vi "pH电极校准.vi"() -> ()   [LabVIEW 2016, in "斯坦道多参数.lvlib"]
uses:
  <vilib>/Utility/miscctls.llb/LVPointTypeDef.ctl
  <vilib>/Analysis/NI_AALBase.lvlib
panel:
  in  "刷新按钮":bool
  out "第三点信号值":dbl
  out "第二点信号值":dbl
  out "第一点信号值":dbl
  out "温度":dbl format="%#.2f"
  out "通讯状态":string
  out "电极状态标志":u16(ring) items=["OK", "第一点校正通过", "第二点校正通过", "校正失败,电极零点超出范围", "校正失败,电极斜率超出范围", "第三点校正通过"]
  in  "三点标液3":u16(ring)=6 caption="标液3" items=["TECH4.00", "TECH7.00", "TECH10.00", "NIST1.68", "NIST4.01", "NIST6.86", "NIST9.18", "NIST12.68"]
  in  "三点标液2":u16(ring)=5 caption="标液2" items=["TECH4.00", "TECH7.00", "TECH10.00", "NIST1.68", "NIST4.01", "NIST6.86", "NIST9.18", "NIST12.68"]
  in  "三点标液1":u16(ring)=4 caption="标液1" items=["TECH4.00", "TECH7.00", "TECH10.00", "NIST1.68", "NIST4.01", "NIST6.86", "NIST9.18", "NIST12.68"]
  out "第三点校准值":dbl
  in  "校准停止":bool
  in  "校准启动":bool
  out "第二点校准值":dbl
  out "第一点校准值":dbl
  out "提示":string
  in  "校准模式":u16(ring) items=["两点校准", "单点校准", "三点校准"]
  out "最小值":sgl format="%#.2f"
  out "最大值":sgl format="%#.2f"
  out "变异系数":dbl format="%#.6f"
  out "standard deviation":dbl caption="标准差" format="%#.2f"
  out "mean":dbl caption="均值" format="%#.2f"
  out "波形图表":dbl(graph) caption="历史曲线"
  out "当前检测值":dbl caption="测量值" format="%#.2f"
  out "标液2":dbl
  out "标液1":dbl
  out "当前信号值":dbl caption="信号值" format="%#.2f"
  out "偏移值补偿":dbl caption="pH偏移修正值" format="%#.2f"
  out "电极斜率":dbl format="%#.6f"
  out "电极零点":dbl format="%#.6f"
  # "酸碱度电极设定"
  # "℃"
  # "mV"
  # "mV"
  # "%"
  # "请选择校准模式:"
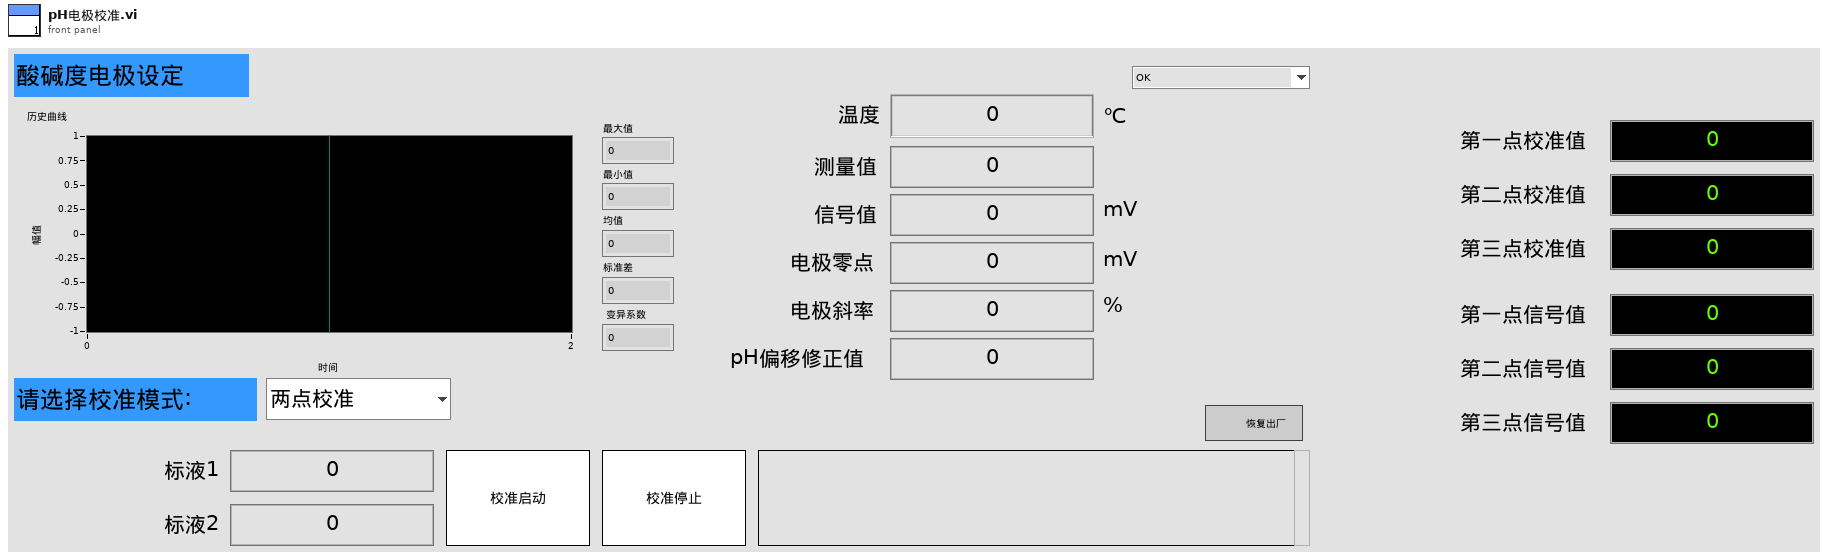
[diagram p1: front panel]
types:
  T1 = typedef "LVPointTypeDef.ctl" = cluster{"Horizontal":i16, "Vertical":i16}
  T2 = cluster{"电极状态标志":u16, "电极型号标志":u16, "酸碱度测量值":sgl, "温度测量值":sgl, "酸碱度信号值":sgl, "温度信号值":sgl, "酸碱度偏移修正值":sgl, "温度偏移修正值":sgl, "手动温度补偿值":sgl, "酸碱度电极零点":sgl, "酸碱度电极斜率":sgl, "第1点标准值记录":sgl, "第1点信号值记录":sgl, "第1点温度值记录":sgl, "第2点标准值记录":sgl, "第2点信号值记录":sgl, "第2点温度值记录":sgl, "命令滤波设定":u16, "温度模式":enum16{"ATC", "MTC"}, "生产批次":u16, "电极序号":u16, "串口地址":u16, "串口波特率":enum16{"9600", "19200", "115200"}, "串口校验位":enum16{"NONE", "ODD", "EVEN"}, "串口停止位":enum16{"1bit", "2bit"}, "第一点标准值":sgl, "第二点标准值":sgl}
  T3 = enum8{"Enabled", "Disabled", "Disabled and Grayed Out"}
  T4 = cluster{"ph":bool, "DO":bool, "Cond":bool, "Turb":bool, "叶绿素a":bool, "藻密度":bool, "ORP":bool}
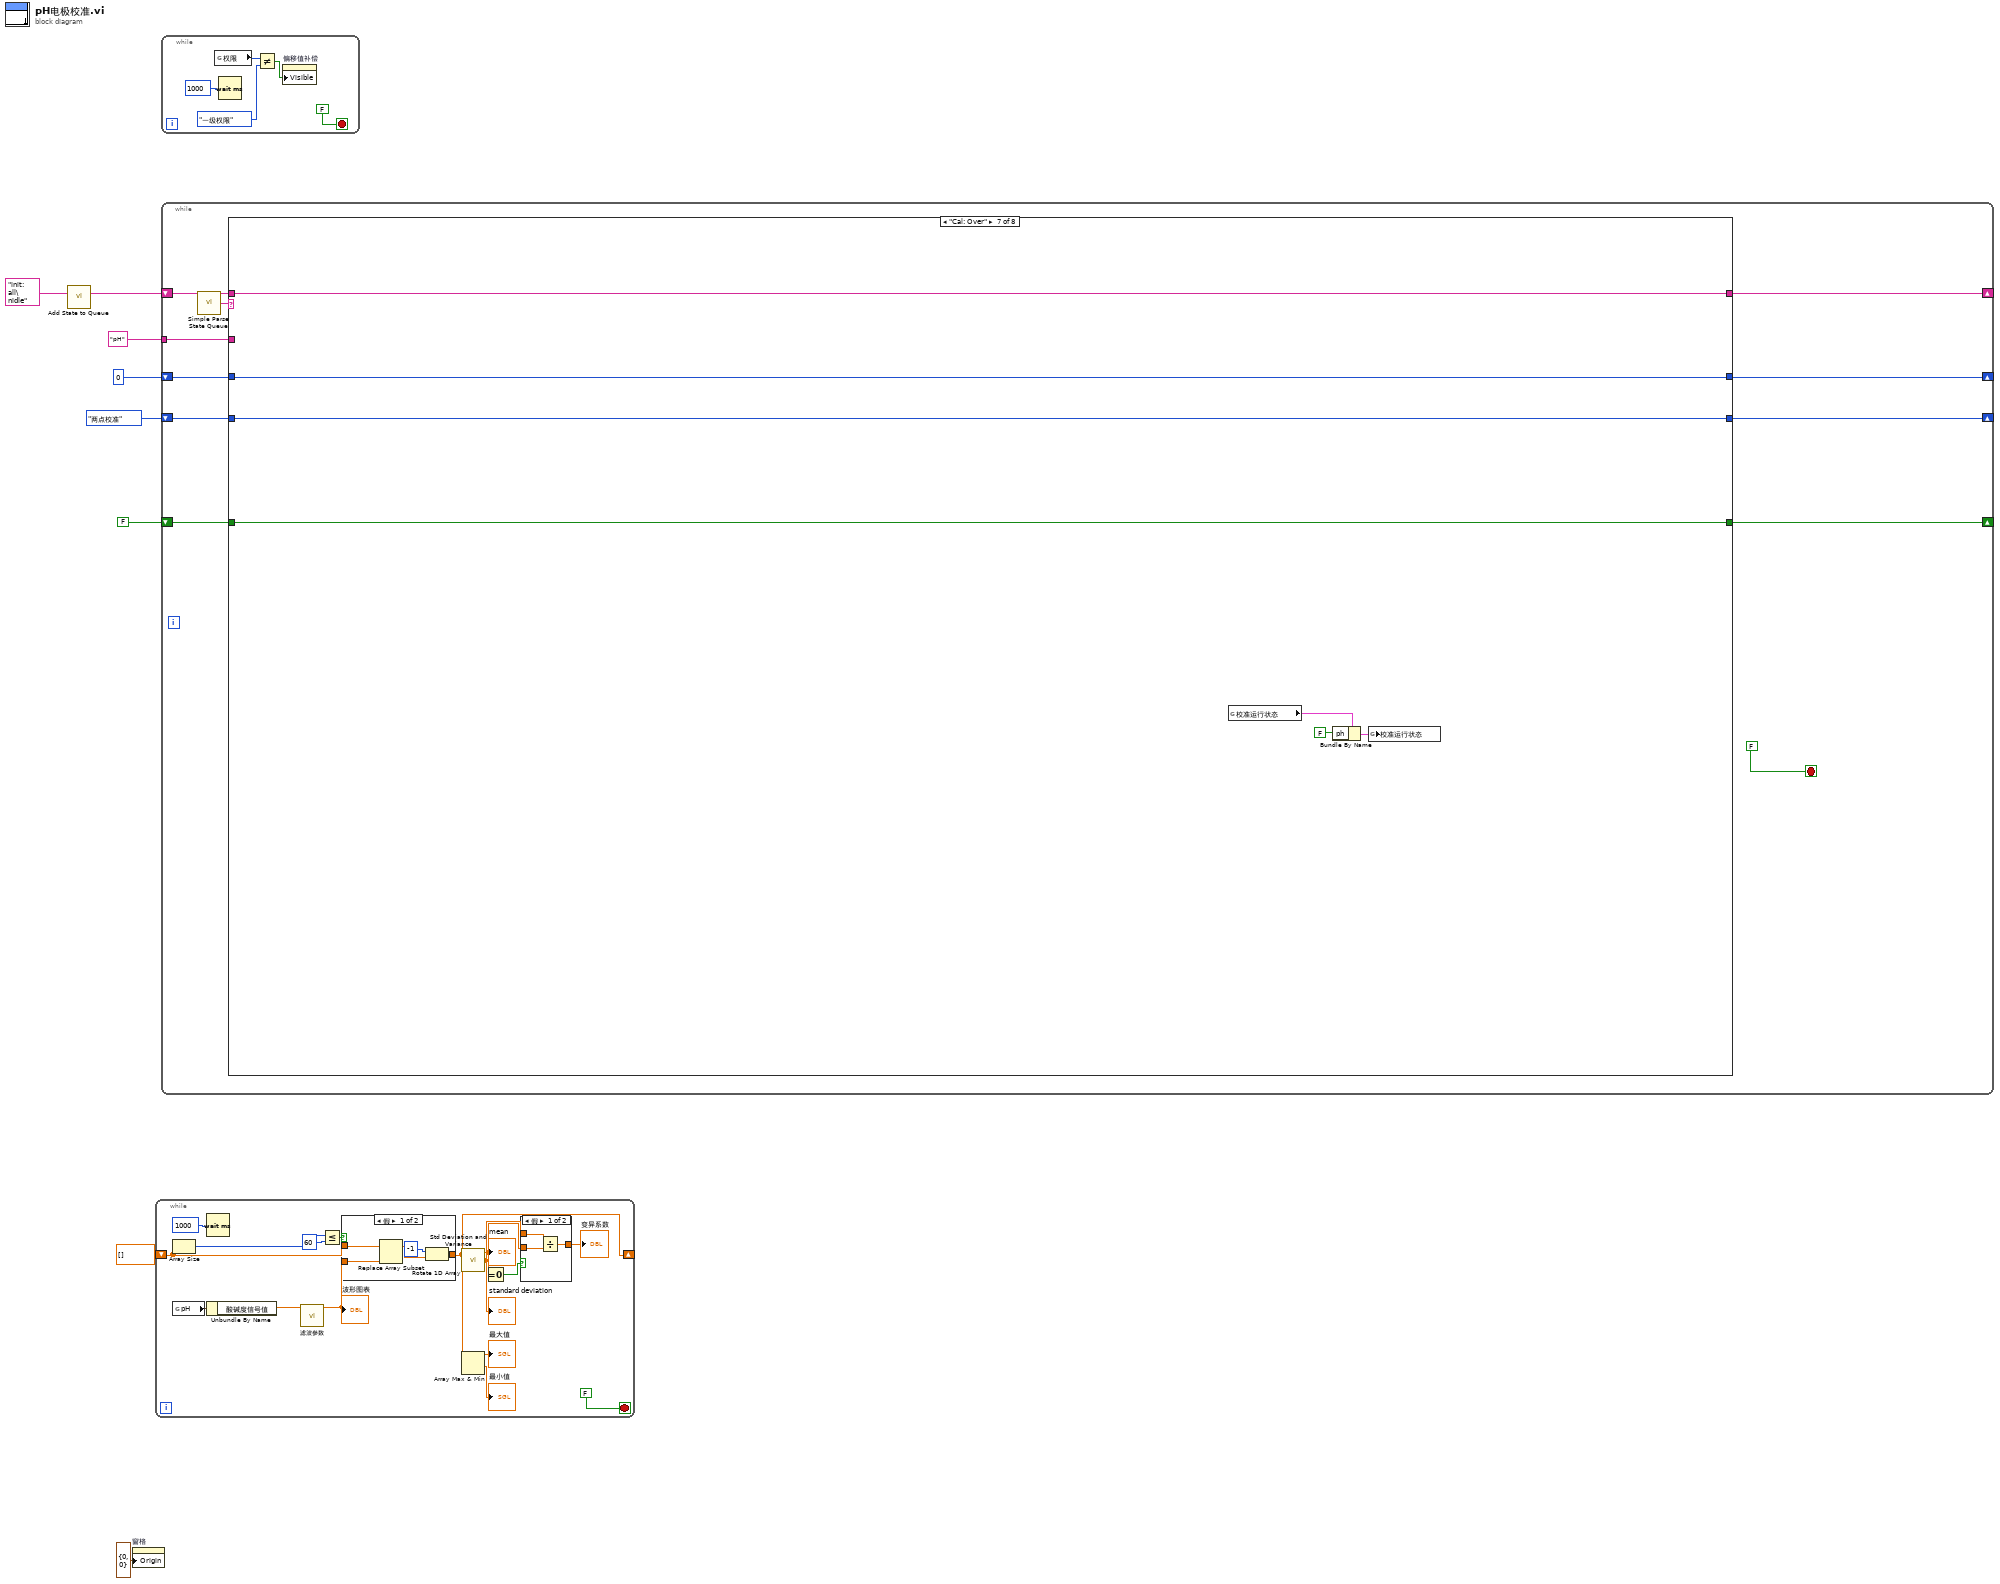
[diagram p0: block diagram]
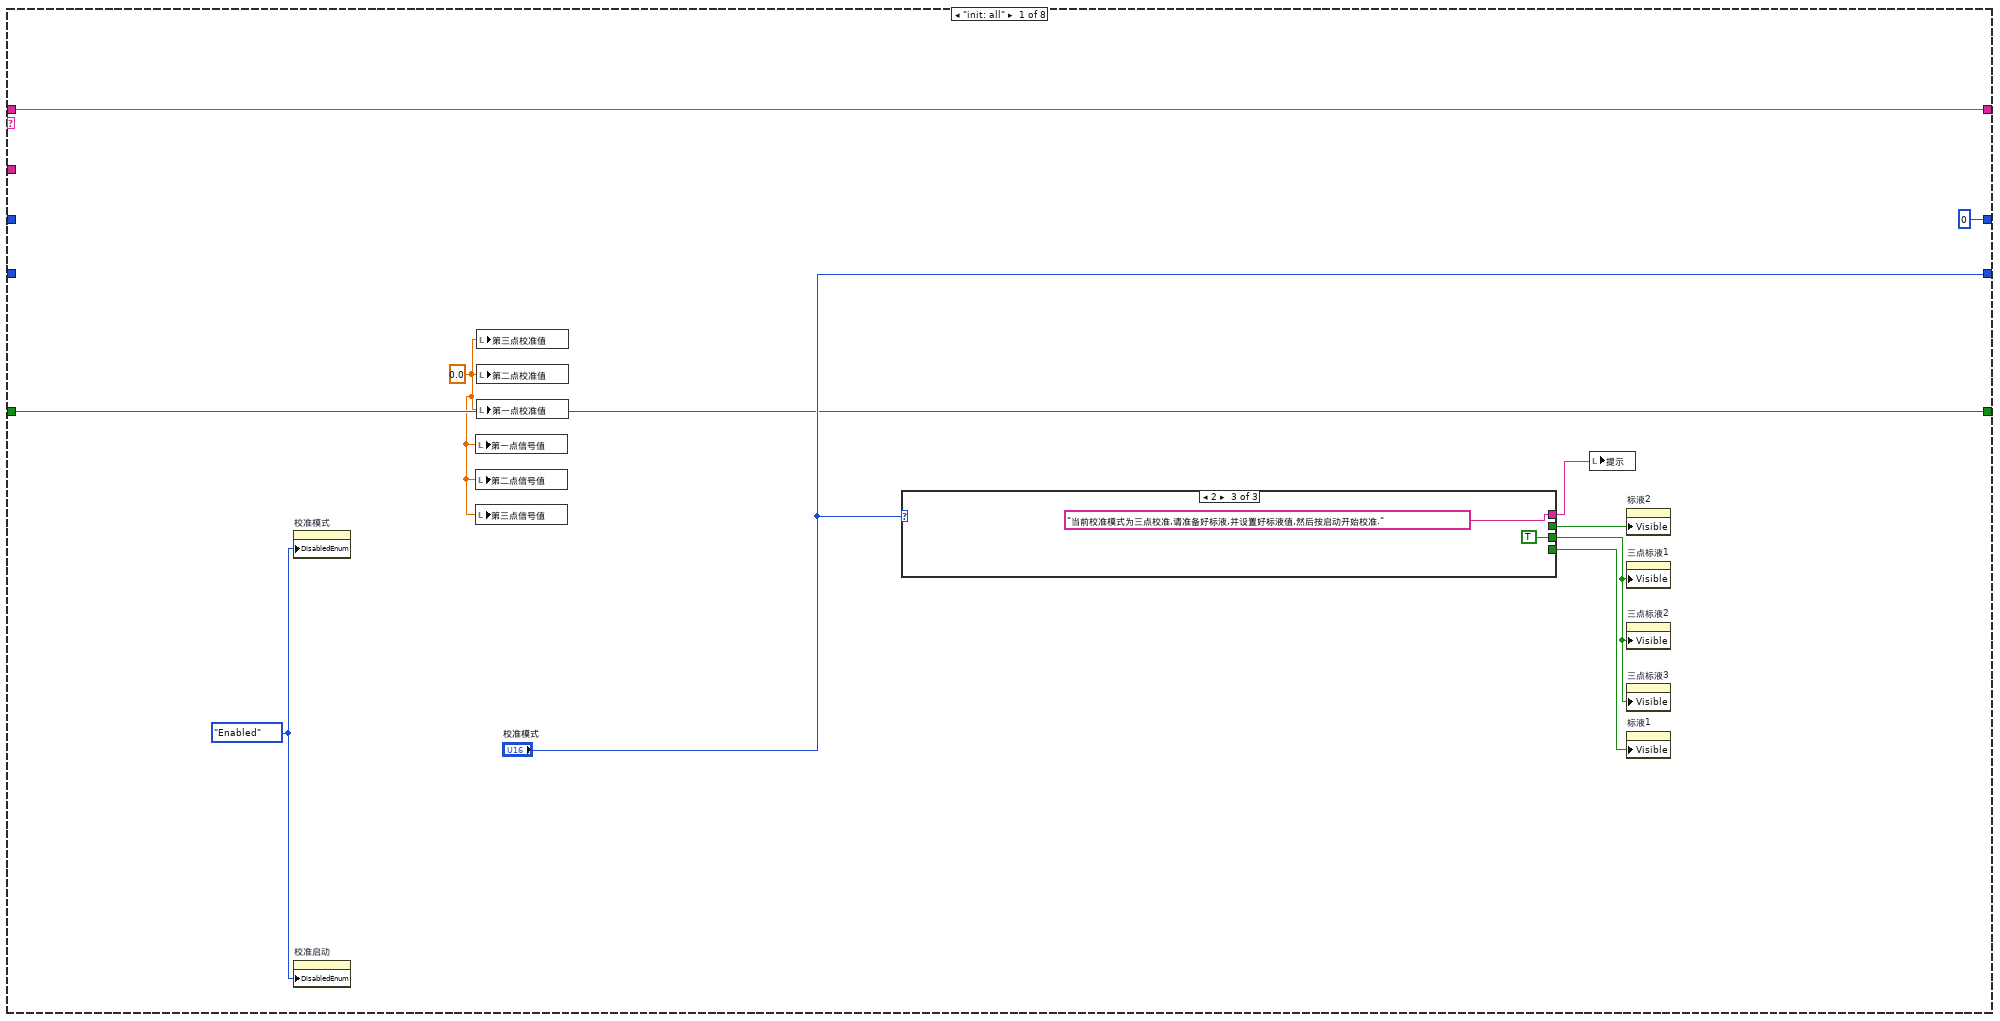
[diagram p2: hidden frame]
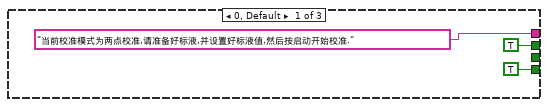
[diagram p3: hidden frame]
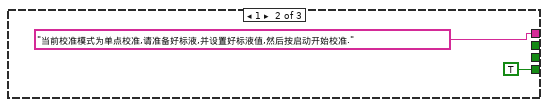
[diagram p4: hidden frame]
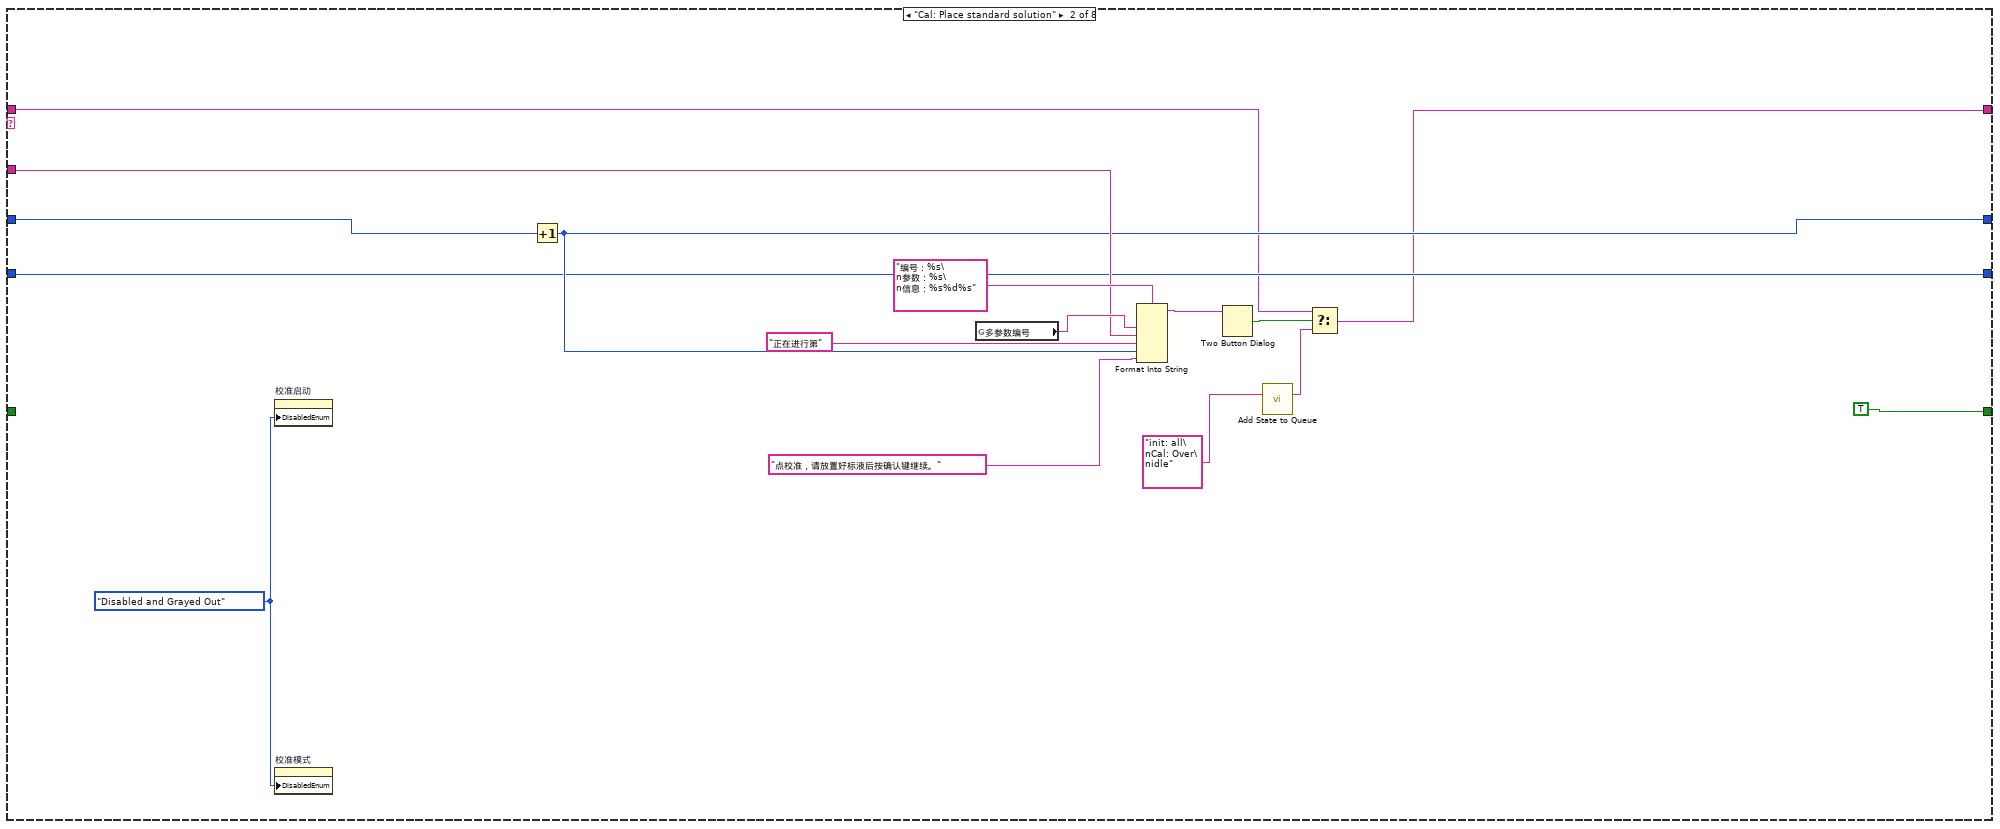
[diagram p5: hidden frame]
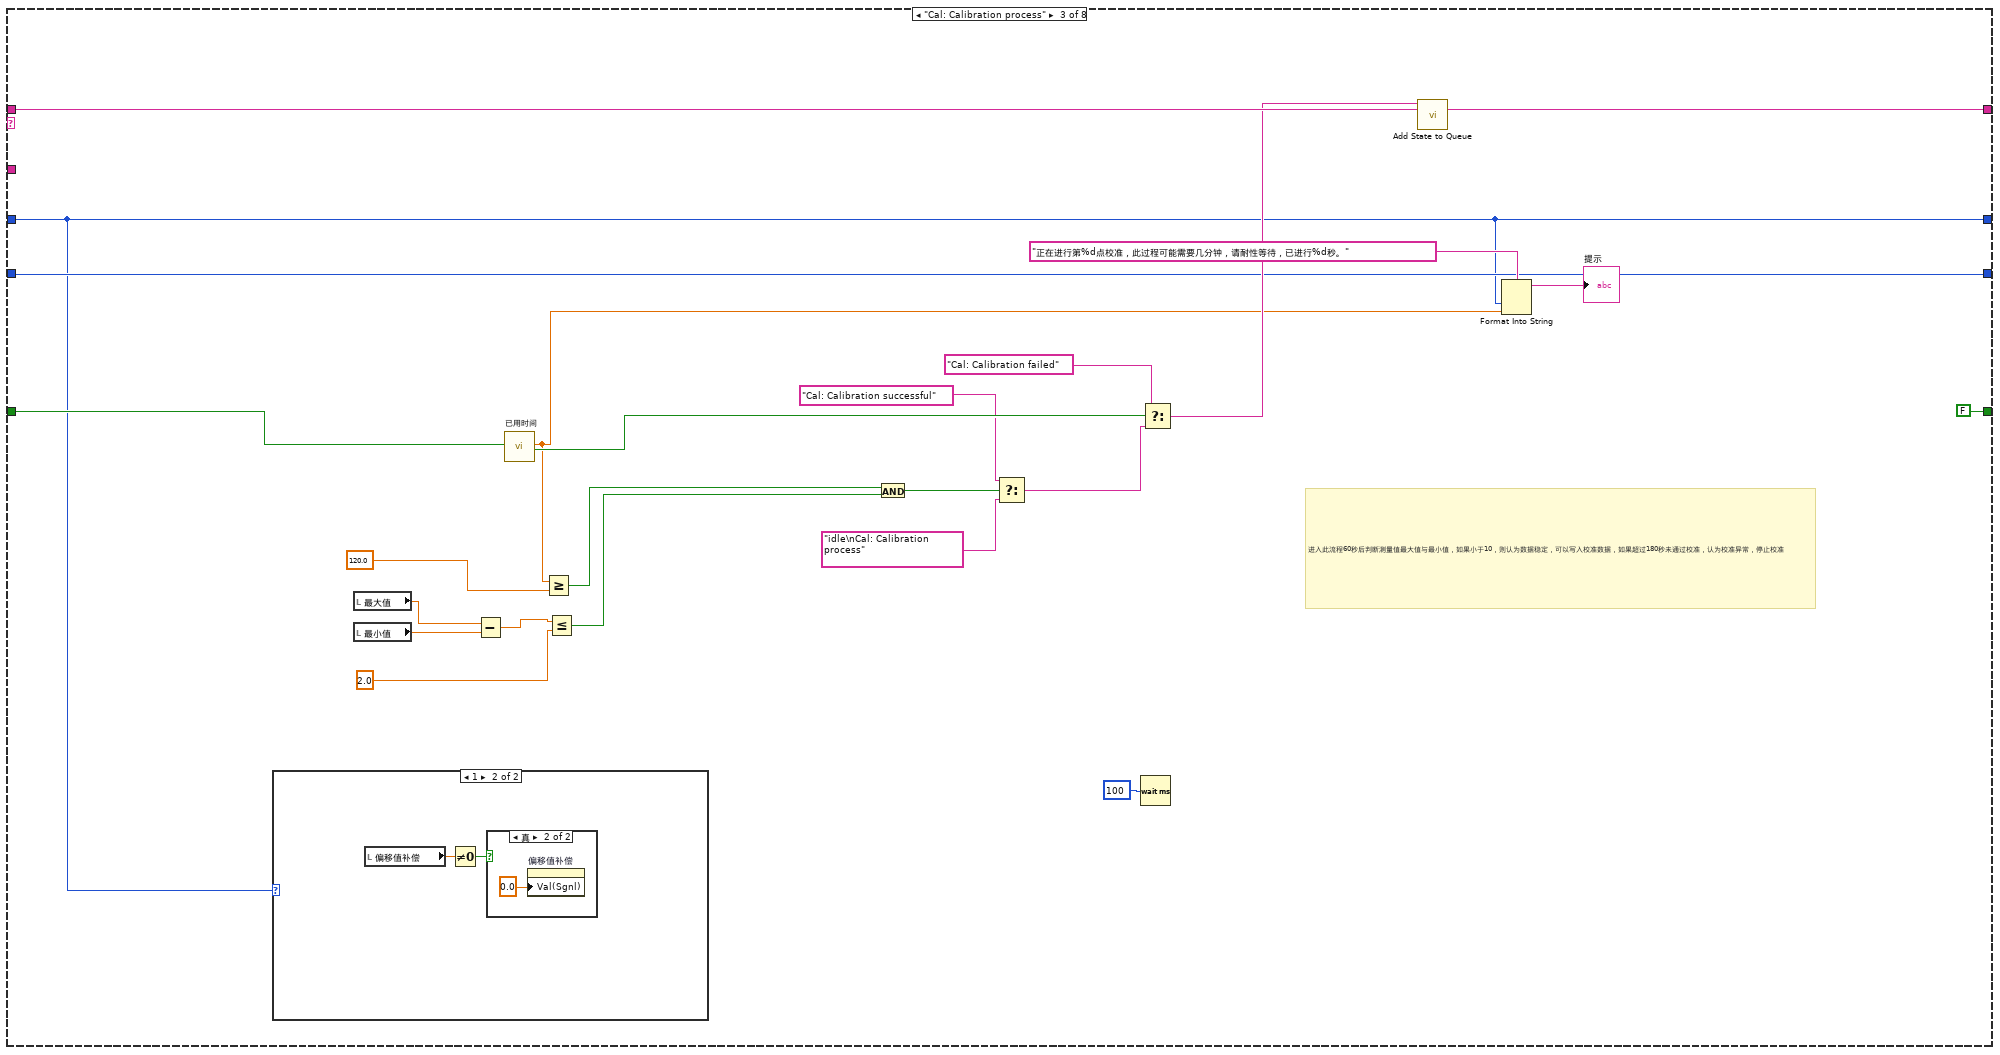
[diagram p6: hidden frame]
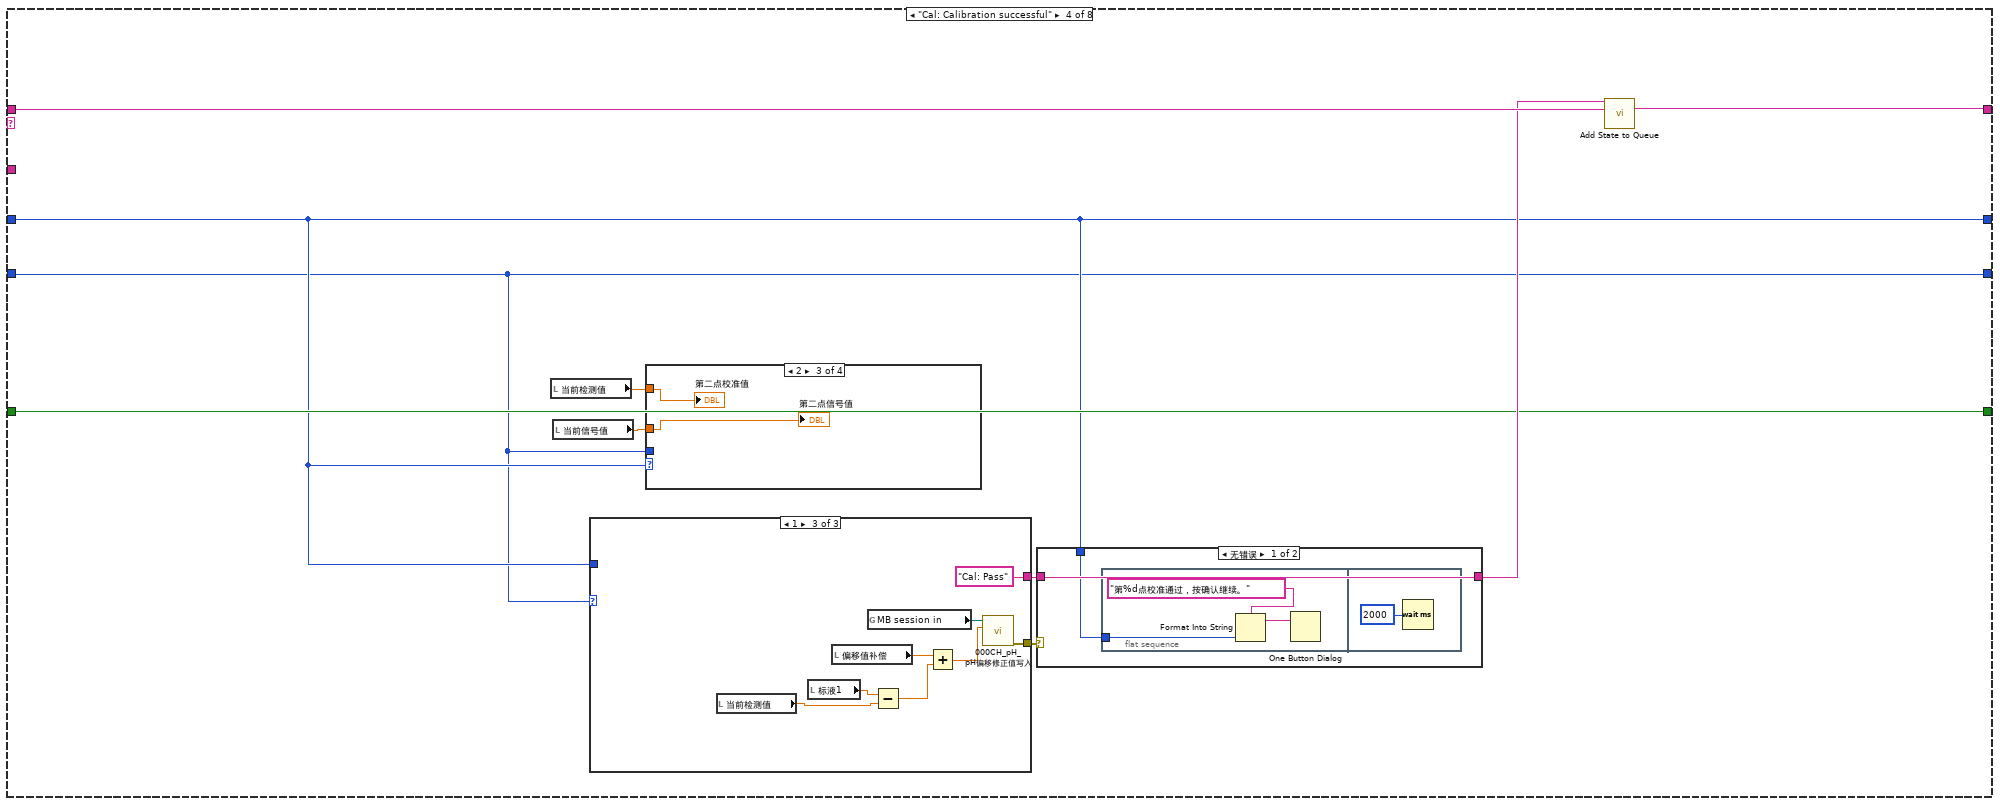
[diagram p9: hidden frame]
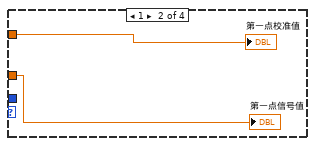
[diagram p11: hidden frame]
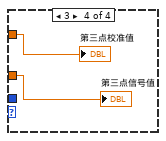
[diagram p12: hidden frame]
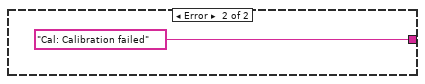
[diagram p13: hidden frame]
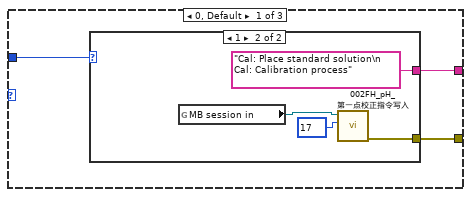
[diagram p14: hidden frame]
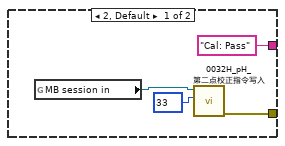
[diagram p15: hidden frame]
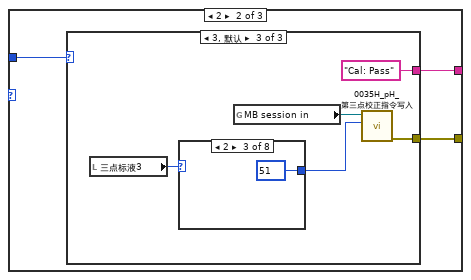
[diagram p16: hidden frame]
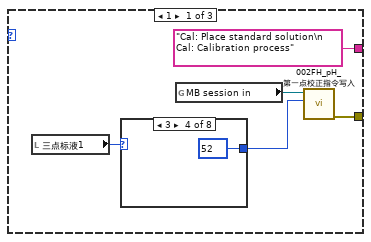
[diagram p17: hidden frame]
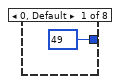
[diagram p18: hidden frame]
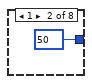
[diagram p19: hidden frame]
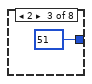
[diagram p20: hidden frame]
diagram:
  n1 = call "Add State to Queue.vi"("State(s) In (\"\")"="init: all\nidle" ("State(s) In (\"\")")) -> ("States Out"=w5:string)  [unwired: 14 in]
  n2 = property on="窗格" class="Pane"("Origin"=T1 {"Horizontal"=0, "Vertical"=0} ("原点")) -> ()  [unwired: 2 in, 2 out]
  n3 = while {
    shift-right: [w16] -> _
    shift-left: sgl[] [] -> [w20]
    stop <- FALSE stop-if-true
    n4 = Array Size(array=w20) -> (size(s)=w22:i32)
    n5 = global read "国弘过程全局变量.vi" "pH"() -> (w17:T2)
    n6 = Wait (ms)(milliseconds to wait=u32 1000 ("等待时间（毫秒）")) -> ()  [unwired: 1 out]
    n7 = Unbundle By Name(w17) -> ("酸碱度信号值"=w10:sgl)
    n8 = call "滤波参数.vi"("x"=w10) -> ("mode"=w9:dbl)  [unwired: 10 in]
    "波形图表" <- w9
    n9 = Less Or Equal?(x=w22, y=60) -> (x <= y?=w21:bool)
    n10 = case shown="假" w21 {
      tunnel: w20 -> [w32 w35]
      tunnel: w9 -> [w30 w34]
      tunnel: [w28 w33] -> w16
      frame False {
        n11 = Replace Array Subset(array=w32, new element=w30) -> (w31:sgl[])  [unwired: 1 in]
        n12 = Rotate 1D Array(1:w31, 2:-1 ("n")) -> (0:w28:sgl[])
      }
      frame True {
        n13 = Insert Into Array(array=w35, new element=w34) -> (w33:sgl[])  [unwired: 1 in]
      }
    }
    n14 = call <vilib>:"Std Deviation and Variance.vi"("X"=w16) -> ("mean"=w12:dbl, "standard deviation"=w11:dbl)  [unwired: 1 in, 1 out]
    "mean" <- w12
    "standard deviation" <- w11
    n15 = Array Max & Min(array=w16) -> (max value=→"最大值":sgl, min value=→"最小值":sgl)  [unwired: 2 out]
    n16 = Equal To 0?(x=w12) -> (x = 0?=w19:bool)
    n17 = case shown="假" w19 {
      tunnel: w11 -> [w27 _]
      tunnel: [w26 _] -> w13
      tunnel: w12 -> [w25 _]
      frame False {
        n18 = Divide(x=w27, y=w25) -> (x/y=w26:dbl)
      }
      frame True {
      }
    }
    "变异系数" <- w13
  }
  n19 = while {
    shift-right: [w43] -> _
    shift-left: w5 -> [w47]
    shift-right: [w40] -> _
    shift-left: 0 -> [w42]
    tunnel: "pH" ("State(s) In (\"\")") -> [w41]
    shift-right: [w38] -> _
    shift-left: enum16{"两点校准", "单点校准", "三点校准"}."两点校准" ("校准模式") -> [w39]
    shift-right: [w36] -> _
    shift-left: FALSE -> [w37]
    stop <- FALSE stop-if-true
    n20 = call "Simple Parse State Queue.vi"("State Queue"=w47) -> ("Remain States"=w44:string, "Next State"=w45:string)  [unwired: 13 in]
    n21 = case shown="\"Cal: Over\"" w45 {
      tunnel: w44 -> [w57 w67 w99 w115 _ _ w260 w270]
      tunnel: [w57 w66 w98 w114 w199 w206 w260 w269] -> w43
      tunnel: w42 -> [_ w76 w82 w109 w202 w215 w259 w267]
      tunnel: w41 -> [_ w77 _ _ w193 w211 _ _]
      tunnel: [0 w74 w82 w109 w202 w215 w259 w268] -> w40
      tunnel: w39 -> [_ w73 w83 w108 w201 w207 w258 w266]
      tunnel: ["校准模式" w73 w83 w108 w201 w207 w258 w266] -> w38
      tunnel: w37 -> [w50 _ w85 w110 w200 w210 w257 w264]
      tunnel: [w50 TRUE FALSE w110 w200 w210 w257 w264] -> w36
      frame "init: all" {
        w49 = T3."Enabled" ("禁用")
        w48 = 0.0 ("第一点校准值")
        n22 = property on="校准模式" class="Ring (严格)"("DisabledEnum"=w49) -> ()  [unwired: 2 in, 2 out]
        n23 = property on="校准启动" class="Bool"("DisabledEnum"=w49) -> ()  [unwired: 2 in, 2 out]
        n24 = local write "第一点信号值"(w48) -> ()
        n25 = local write "第二点信号值"(w48) -> ()
        n26 = local write "第三点信号值"(w48) -> ()
        n27 = local write "第三点校准值"(w48) -> ()
        n28 = local write "第二点校准值"(w48) -> ()
        n29 = local write "第一点校准值"(w48) -> ()
        n30 = case shown="2" "校准模式" {
          tunnel: ["当前校准模式为两点校准,请准备好标液,并设置好标液值,然后按启动开始校准." ("提示") "当前校准模式为单点校准,请准备好标液,并设置好标液值,然后按启动开始校准." ("提示") "当前校准模式为三点校准,请准备好标液,并设置好标液值,然后按启动开始校准." ("提示")] -> w52
          tunnel: [TRUE ("可见") _ _] -> w56
          tunnel: [TRUE ("可见") TRUE ("可见") _] -> w54
          tunnel: [_ _ TRUE ("可见")] -> w55
          frame 0, Default {
          }
          frame 1 {
          }
          frame 2 {
          }
        }
        n31 = local write "提示"(w52) -> ()
        n32 = property on="标液2" class="DigNum (严格)"("Visible"=w56) -> ()  [unwired: 2 in, 2 out]
        n33 = property on="三点标液1" class="Ring (严格)"("Visible"=w55) -> ()  [unwired: 2 in, 2 out]
        n34 = property on="三点标液2" class="Ring (严格)"("Visible"=w55) -> ()  [unwired: 2 in, 2 out]
        n35 = property on="三点标液3" class="Ring (严格)"("Visible"=w55) -> ()  [unwired: 2 in, 2 out]
        n36 = property on="标液1" class="DigNum (严格)"("Visible"=w54) -> ()  [unwired: 2 in, 2 out]
      }
      frame "Cal: Place standard solution" {
        w71 = T3."Disabled and Grayed Out" ("禁用")
        n37 = property on="校准启动" class="Bool"("DisabledEnum"=w71) -> ()  [unwired: 2 in, 2 out]
        n38 = property on="校准模式" class="Ring (严格)"("DisabledEnum"=w71) -> ()  [unwired: 2 in, 2 out]
        n39 = Increment(x=w76) -> (x+1=w74:i32)
        n40 = global read "多参数全局变量.vi" "多参数编号"() -> (w79:string)
        n41 = Format Into String(format string="编号：%s\n参数：%s\n信息：%s%d%s" ("格式字符串"), w79, w77, "正在进行第" ("消息"), w74, "点校准，请放置好标液后按确认键继续。" ("消息")) -> (resulting string=w70:string)  [unwired: 2 in, 1 out]
        n42 = Two Button Dialog(message=w70) -> (T button?=w69:bool)  [unwired: 2 in]
        n43 = call "Add State to Queue.vi"("State(s) In (\"\")"="init: all\nCal: Over\nidle" ("State(s) In (\"\")")) -> ("States Out"=w68:string)  [unwired: 14 in]
        n44 = Select(t=w67, s=w69, f=w68) -> (s? t:f=w66:string)
      }
      frame "Cal: Calibration process" {
        # "进入此流程60秒后判断测量值最大值与最小值，如果小于10，则认为数据稳定，可以写入校准数据，如果超过180秒未通过校准，认为校准异常，停止校准"
        n45 = case shown="1" w82 {
          frame 0, Default {
          }
          frame 1 {
            n46 = local read "偏移值补偿"() -> (w105:dbl)
            n47 = Not Equal To 0?(x=w105) -> (x != 0?=w106:bool)
            n48 = case shown="真" w106 {
              frame False {
              }
              frame True {
                n49 = property on="偏移值补偿" class="DigNum (严格)"("Val(Sgnl)"=0.0 ("值(信号)")) -> ()  [unwired: 2 in, 2 out]
              }
            }
          }
        }
        n50 = local read "最大值"() -> (w103:sgl)
        n51 = local read "最小值"() -> (w102:sgl)
        n52 = Subtract(x=w103, y=w102) -> (x-y=w104:sgl)
        n53 = call "已用时间"("Reset"=w85) -> ("Elapsed Time (s)"=w81:dbl, "Time has Elapsed"=w100:bool)  [unwired: 11 in, 6 out]
        n54 = Greater Or Equal?(x=w81, y=120.0) -> (x >= y?=w95:bool)
        n55 = Less Or Equal?(x=w104, y=2.0) -> (x <= y?=w91:bool)
        n56 = And(x=w95, y=w91) -> (x .and. y?=w92:bool)
        n57 = Select(t="Cal: Calibration successful" ("State(s) In (\"\")"), s=w92, f="idle\nCal: Calibration process" ("State(s) In (\"\")")) -> (s? t:f=w90:string)
        n58 = Wait (ms)(milliseconds to wait=u32 100 ("等待时间（毫秒）")) -> ()  [unwired: 1 out]
        n59 = Select(t="Cal: Calibration failed" ("State(s) In (\"\")"), s=w100, f=w90) -> (s? t:f=w89:string)
        n60 = call "Add State to Queue.vi"("State(s) In Front (\"\")"=w89, "State(s) In (\"\")"=w99) -> ("States Out"=w98:string)  [unwired: 13 in]
        n61 = Format Into String(format string="正在进行第%d点校准，此过程可能需要几分钟，请耐性等待，已进行%d秒。" ("格式字符串"), w82, w81) -> (resulting string=→"提示":string)  [unwired: 2 in, 1 out]
      }
      frame "Cal: Calibration successful" {
        n62 = local read "当前检测值"() -> (w111:dbl)
        n63 = local read "当前信号值"() -> (w112:dbl)
        n64 = case shown="1" w108 {
          tunnel: [w133 w144 w186] -> w117
          tunnel: [w132 w142 "Cal: Pass" ("State(s) In (\"\")")] -> w116
          tunnel: w109 -> [w131 w143 _]
          frame 0, Default {
            n65 = case shown="1" w131 {
              tunnel: [w134 w139] -> w133
              tunnel: ["Cal: Pass" ("State(s) In (\"\")") "Cal: Place standard solution\n Cal: Calibration process" ("State(s) In (\"\")")] -> w132
              frame 2, Default {
                n66 = global read "多参数全局变量.vi" "MB session in"() -> (w136:refnum<class "MB_Master.lvclass">)
                n67 = call "0032H_pH_第二点校正指令写入.vi"("数值"=u16 33, "MB session in"=w136) -> ("error out"=w134:errorcluster)  [unwired: 8 in, 1 out]
              }
              frame 1 {
                n68 = global read "多参数全局变量.vi" "MB session in"() -> (w141:refnum<class "MB_Master.lvclass">)
                n69 = call "002FH_pH_第一点校正指令写入.vi"("数值"=u16 17, "MB session in"=w141) -> ("error out"=w139:errorcluster)  [unwired: 8 in, 1 out]
              }
            }
          }
          frame 2 {
            n70 = case shown="3, 默认" w143 {
              tunnel: [w146 w159 w172] -> w144
              tunnel: ["Cal: Place standard solution\n Cal: Calibration process" ("State(s) In (\"\")") "Cal: Place standard solution\n Cal: Calibration process" ("State(s) In (\"\")") "Cal: Pass" ("State(s) In (\"\")")] -> w142
              frame 1 {
                n71 = local read "三点标液1"() -> (w148:u16)
                n72 = case shown="3" w148 {
                  tunnel: [u16 49 ("数值") u16 50 ("数值") u16 51 ("数值") u16 52 ("数值") u16 53 ("数值") u16 54 ("数值") u16 55 ("数值") u16 56 ("数值")] -> w147
                  frame 0, Default {
                  }
                  frame 1 {
                  }
                  frame 2 {
                  }
                  frame 3 {
                  }
                  frame 4 {
                  }
                  frame 5 {
                  }
                  frame 6 {
                  }
                  frame 7 {
                  }
                }
                n73 = global read "多参数全局变量.vi" "MB session in"() -> (w149:refnum<class "MB_Master.lvclass">)
                n74 = call "002FH_pH_第一点校正指令写入.vi"("数值"=w147, "MB session in"=w149) -> ("error out"=w146:errorcluster)  [unwired: 8 in, 1 out]
              }
              frame 2 {
                n75 = local read "三点标液2"() -> (w161:u16)
                n76 = case shown="7" w161 {
                  tunnel: [u16 49 ("数值") u16 50 ("数值") u16 51 ("数值") u16 52 ("数值") u16 53 ("数值") u16 54 ("数值") u16 55 ("数值") u16 56 ("数值")] -> w160
                  frame 0, Default {
                  }
                  frame 1 {
                  }
                  frame 2 {
                  }
                  frame 3 {
                  }
                  frame 4 {
                  }
                  frame 5 {
                  }
                  frame 6 {
                  }
                  frame 7 {
                  }
                }
                n77 = global read "多参数全局变量.vi" "MB session in"() -> (w162:refnum<class "MB_Master.lvclass">)
                n78 = call "0032H_pH_第二点校正指令写入.vi"("数值"=w160, "MB session in"=w162) -> ("error out"=w159:errorcluster)  [unwired: 8 in, 1 out]
              }
              frame 3, Default {
                n79 = local read "三点标液3"() -> (w174:u16)
                n80 = case shown="2" w174 {
                  tunnel: [u16 49 ("数值") u16 50 ("数值") u16 51 ("数值") u16 52 ("数值") u16 53 ("数值") u16 54 ("数值") u16 55 ("数值") u16 56 ("数值")] -> w173
                  frame 0, Default {
                  }
                  frame 1 {
                  }
                  frame 2 {
                  }
                  frame 3 {
                  }
                  frame 4 {
                  }
                  frame 5 {
                  }
                  frame 6 {
                  }
                  frame 7 {
                  }
                }
                n81 = global read "多参数全局变量.vi" "MB session in"() -> (w175:refnum<class "MB_Master.lvclass">)
                n82 = call "0035H_pH_第三点校正指令写入.vi"("数值"=w173, "MB session in"=w175) -> ("error out"=w172:errorcluster)  [unwired: 8 in, 1 out]
              }
            }
          }
          frame 1 {
            n83 = local read "当前检测值"() -> (w184:dbl)
            n84 = local read "标液1"() -> (w191:dbl)
            n85 = local read "偏移值补偿"() -> (w187:dbl)
            n86 = global read "多参数全局变量.vi" "MB session in"() -> (w190:refnum<class "MB_Master.lvclass">)
            n87 = Subtract(x=w191, y=w184) -> (x-y=w189:dbl)
            n88 = Add(x=w187, y=w189) -> (x+y=w188:dbl)
            n89 = call "000CH_pH_pH偏移修正值写入.vi"("数值"=w188, "MB session in"=w190) -> ("error out"=w186:errorcluster)  [unwired: 8 in, 1 out]
          }
        }
        n90 = case shown="2" w109 {
          tunnel: w112 -> [_ w119 w120 w122]
          tunnel: w111 -> [_ w118 w121 w123]
          tunnel: w108 -> [_ _ _ _]
          frame 0, Default {
          }
          frame 1 {
            "第一点校准值" <- w118
            "第一点信号值" <- w119
          }
          frame 2 {
            "第二点校准值" <- w121
            "第二点信号值" <- w120
          }
          frame 3 {
            "第三点校准值" <- w123
            "第三点信号值" <- w122
          }
        }
        n91 = case shown="无错误" w117 {
          tunnel: w116 -> [w125 _]
          tunnel: [w125 "Cal: Calibration failed" ("State(s) In (\"\")")] -> w113
          tunnel: w109 -> [w124 _]
          frame No Error {
            n92 = flat-sequence {
              tunnel: w124 -> [w126]
              frame #0 {
                n93 = Format Into String(format string="第%d点校准通过，按确认继续。" ("格式字符串"), w126) -> (resulting string=w128:string)  [unwired: 2 in, 1 out]
                n94 = One Button Dialog(message=w128) -> ()  [unwired: 1 in, 1 out]
              }
              frame #1 {
                n95 = Wait (ms)(milliseconds to wait=u32 2000 ("等待时间（毫秒）")) -> ()  [unwired: 1 out]
              }
            }
          }
          frame Error {
          }
        }
        n96 = call "Add State to Queue.vi"("State(s) In Front (\"\")"=w113, "State(s) In (\"\")"=w115) -> ("States Out"=w114:string)  [unwired: 13 in]
      }
      frame "Cal: Calibration failed" {
        n97 = global read "多参数全局变量.vi" "多参数编号"() -> (w196:string)
        n98 = call "Add State to Queue.vi"("State(s) In (\"\")"="init: all\nCal: Over\nidle" ("State(s) In (\"\")")) -> ("States Out"=w199:string)  [unwired: 14 in]
        n99 = Format Into String(format string="编号：%s\n参数：%s\n信息：%s" ("格式字符串"), w196, w193, "校准失败！" ("消息")) -> (resulting string=w195:string)  [unwired: 2 in, 1 out]
        n100 = One Button Dialog(message=w195) -> ()  [unwired: 1 in, 1 out]
        n101 = call "校准日志.vi"("table"="校准记录", "日志信息"=w195) -> ()  [unwired: 9 in, 1 out]
      }
      frame "Cal: Pass" {
        n102 = flat-sequence {
          tunnel: [w220] -> w208
          tunnel: w207 -> [w219]
          tunnel: [w218] -> w205
          tunnel: [w217] -> w204
          frame #0 {
            n103 = Wait (ms)(milliseconds to wait=u32 3000 ("等待时间（毫秒）")) -> ()  [unwired: 1 out]
          }
          frame #1 {
            n104 = global read "国弘过程全局变量.vi" "pH"() -> (w221:T2)
            n105 = Unbundle By Name(w221) -> ("电极状态标志"=w222:u16, "酸碱度电极零点"=w218:sgl, "酸碱度电极斜率"=w217:sgl)
            n106 = case shown="0, 默认" w219 {
              tunnel: [w224 w239 w256] -> w220
              tunnel: w222 -> [w223 w238 _]
              frame 0, Default {
                n107 = case shown="2" w223 {
                  selector: w223 -> [_ _ w235]
                  tunnel: ["校准异常，校准未完成。" ("格式字符串") w233 w234] -> w224
                  frame 0, Default {
                  }
                  frame 2 {
                    n108 = local read "第一点校准值"() -> (w231:dbl)
                    n109 = local read "第一点信号值"() -> (w232:dbl)
                    n110 = local read "第二点校准值"() -> (w228:dbl)
                    n111 = local read "第二点信号值"() -> (w227:dbl)
                    n112 = local read "标液1"() -> (w229:dbl)
                    n113 = local read "标液2"() -> (w226:dbl)
                    n114 = Format Into String(format string="校准结果：\n第一点校准值=%#.2f，第一点信号值=%#.2f mV，第一点标准值=%#.2f；\n第二点校准值=%#.2f，第二点信号值=%#.2f mV，第二点标准值=%#.2f。" ("提示"), w231, w232, w229, w228, w227, w226) -> (resulting string=w233:string)  [unwired: 2 in, 1 out]
                  }
                  frame 3, 4 {
                    n115 = case shown="4" w235 {
                      tunnel: ["校正失败，电极零点超出范围" "校正失败，电极斜率超出范围"] -> w234
                      frame 3, Default {
                      }
                      frame 4 {
                      }
                    }
                  }
                }
              }
              frame 2 {
                n116 = case shown="5" w238 {
                  tunnel: ["校准异常，校准未完成。" ("格式字符串") w251] -> w239
                  frame 0, Default {
                  }
                  frame 5 {
                    n117 = local read "第一点校准值"() -> (w250:dbl)
                    n118 = local read "第一点信号值"() -> (w248:dbl)
                    n119 = local read "第二点校准值"() -> (w246:dbl)
                    n120 = local read "第二点信号值"() -> (w245:dbl)
                    n121 = local read "第三点校准值"() -> (w243:dbl)
                    n122 = local read "第三点信号值"() -> (w242:dbl)
                    n123 = property on="三点标液1" class="Ring (严格)"() -> ("RingText.Text"=w247:string)  [unwired: 2 in, 2 out]
                    n124 = property on="三点标液2" class="Ring (严格)"() -> ("RingText.Text"=w244:string)  [unwired: 2 in, 2 out]
                    n125 = property on="三点标液3" class="Ring (严格)"() -> ("RingText.Text"=w241:string)  [unwired: 2 in, 2 out]
                    n126 = Format Into String(format string="校准结果：\n第一点校准值=%#.2f，第一点信号值=%#.2f mV，第一点标准值=%s；\n第二点校准值=%#.2f，第二点信号值=%#.2f mV，第二点标准值=%s；\n第三点校准值=%#.2f，第三点信号值=%#.2f mV，第三点标准值=%s。" ("提示"), w250, w248, w247, w246, w245, w244, w243, w242, w241) -> (resulting string=w251:string)  [unwired: 2 in, 1 out]
                  }
                }
              }
              frame 1 {
                n127 = local read "第一点校准值"() -> (w255:dbl)
                n128 = local read "第一点信号值"() -> (w253:dbl)
                n129 = local read "标液1"() -> (w252:dbl)
                n130 = Format Into String(format string="校准结果：\n校准值=%#.2f，信号值=%#.2f，标准值=%#.2f。" ("提示"), w255, w253, w252) -> (resulting string=w256:string)  [unwired: 2 in, 1 out]
              }
            }
          }
        }
        n131 = call "Add State to Queue.vi"("State(s) In (\"\")"="init: all\nCal: Over\nidle" ("State(s) In (\"\")")) -> ("States Out"=w206:string)  [unwired: 14 in]
        n132 = global read "多参数全局变量.vi" "多参数编号"() -> (w212:string)
        n133 = Format Into String(format string="编号：%s\n参数：%s\n信息：%s\n电极零点=%#.2f，电极斜率=%#.2f%%。" ("格式字符串"), w212, w211, w208, w205, w204) -> (resulting string=w209:string)  [unwired: 2 in, 1 out]
        n134 = One Button Dialog(message=w209) -> ()  [unwired: 1 in, 1 out]
        n135 = call "校准日志.vi"("table"="校准记录", "日志信息"=w209) -> ()  [unwired: 9 in, 1 out]
      }
      frame "Cal: Over" {
        n136 = global read "多参数全局变量.vi" "校准运行状态"() -> (w262:T4)
        n137 = Bundle By Name(cluster=w262, "ph"=FALSE) -> (w263:T4)
        n138 = global write "多参数全局变量.vi" "校准运行状态"(w263) -> ()
      }
      frame "idle", Default {
        n139 = event shown="[10] \"校准启动\": 值改变" {
          selector: _ -> [_ _ _ _ _ _ _ _ _ _ _ _]
          dyn-events: _ -> [_ _ _ _ _ _ _ _ _ _ _ _]
          timeout: 10 -> [_ _ _ _ _ _ _ _ _ _ _ _]
          tunnel: [_ _ _ _ _ _ w355 w365 w371 _ _ _] -> _
          tunnel: w270 -> [w287 w291 w292 w314 w328 w346 w360 w361 w367 w375 w386 _]
          tunnel: [w286 w290 w293 w315 w329 w347 w359 w362 w368 w374 w385 w388] -> w269
          tunnel: [w285 w288 w294 w316 w330 w349 w358 w363 w369 w373 w383 w389] -> w268
          tunnel: w267 -> [w285 w288 w294 w316 w330 w349 w358 w363 w369 w373 w383 w389]
          event Timeout {
            n140 = event-data() -> ()  [unwired: 1 in, 3 out]
            n141 = global read "国弘过程全局变量.vi" "pH"() -> (w284:T2)
            n142 = Unbundle By Name(w284) -> ("电极状态标志"=→"电极状态标志":u16, "酸碱度电极零点"=→"电极零点":sgl, "酸碱度电极斜率"=→"电极斜率":sgl, "酸碱度偏移修正值"=→"偏移值补偿":sgl, "酸碱度信号值"=→"当前信号值":sgl, "第一点标准值"=→"标液1":sgl, "第二点标准值"=→"标液2":sgl, "酸碱度测量值"=→"当前检测值":sgl, "温度测量值"=→"温度":sgl)  [unwired: 1 out]
            n143 = global read "多参数全局变量.vi" "ph通讯状态"() -> (w273:bool)
            n144 = property on="通讯状态" class="Str"("Blinking"=TRUE ("闪烁"), "Text.BG Color"=u32 16711680, "Visible"=w273) -> ()  [unwired: 2 in, 2 out]
            n145 = call "Add State to Queue.vi"("State(s) In (\"\")"=w287) -> ("States Out"=w286:string)  [unwired: 14 in]
            "通讯状态" <- "通讯异常" ("当前串口")
          }
          event "校准模式": Value Change {
            n146 = event-data() -> ()  [unwired: 1 in, 6 out]
            n147 = call "Add State to Queue.vi"("State(s) In (\"\")"=w291, "State(s) At Back (\"\")"="init: all\nidle" ("State(s) In (\"\")")) -> ("States Out"=w290:string)  [unwired: 13 in]
          }
          event "三点标液1": Value Change {
            n148 = event-data() -> ("NewVal"=w295:u16)  [unwired: 1 in, 5 out]
            n149 = case shown="1" w295 {
              frame 0, Default {
                w296 = u16 0 items=["TECH4.00", "TECH7.00", "TECH10.00", "NIST1.68", "NIST4.01", "NIST6.86", "NIST9.18", "NIST12.68"] ("标液2")
                w297 = u16 2 items=["TECH4.00", "TECH7.00", "TECH10.00", "NIST1.68", "NIST4.01", "NIST6.86", "NIST9.18", "NIST12.68"] ("标液3")
                w298 = u16 1 items=["TECH4.00", "TECH7.00", "TECH10.00", "NIST1.68", "NIST4.01", "NIST6.86", "NIST9.18", "NIST12.68"] ("标液2")
                n150 = local write "三点标液3"(w297) -> ()
                n151 = local write "三点标液2"(w298) -> ()
                n152 = local write "三点标液1"(w296) -> ()
              }
              frame 1 {
                w299 = u16 0 items=["TECH4.00", "TECH7.00", "TECH10.00", "NIST1.68", "NIST4.01", "NIST6.86", "NIST9.18", "NIST12.68"] ("标液2")
                w300 = u16 2 items=["TECH4.00", "TECH7.00", "TECH10.00", "NIST1.68", "NIST4.01", "NIST6.86", "NIST9.18", "NIST12.68"] ("标液3")
                w301 = u16 1 items=["TECH4.00", "TECH7.00", "TECH10.00", "NIST1.68", "NIST4.01", "NIST6.86", "NIST9.18", "NIST12.68"] ("标液2")
                n153 = local write "三点标液3"(w300) -> ()
                n154 = local write "三点标液2"(w301) -> ()
                n155 = local write "三点标液1"(w299) -> ()
              }
              frame 2 {
                w302 = u16 2 items=["TECH4.00", "TECH7.00", "TECH10.00", "NIST1.68", "NIST4.01", "NIST6.86", "NIST9.18", "NIST12.68"] ("标液2")
                w303 = u16 0 items=["TECH4.00", "TECH7.00", "TECH10.00", "NIST1.68", "NIST4.01", "NIST6.86", "NIST9.18", "NIST12.68"] ("标液3")
                w304 = u16 1 items=["TECH4.00", "TECH7.00", "TECH10.00", "NIST1.68", "NIST4.01", "NIST6.86", "NIST9.18", "NIST12.68"] ("标液2")
                n156 = local write "三点标液3"(w303) -> ()
                n157 = local write "三点标液2"(w304) -> ()
                n158 = local write "三点标液1"(w302) -> ()
              }
              frame 3 {
                w305 = u16 3 items=["TECH4.00", "TECH7.00", "TECH10.00", "NIST1.68", "NIST4.01", "NIST6.86", "NIST9.18", "NIST12.68"] ("标液2")
                w306 = u16 5 items=["TECH4.00", "TECH7.00", "TECH10.00", "NIST1.68", "NIST4.01", "NIST6.86", "NIST9.18", "NIST12.68"] ("标液3")
                w307 = u16 4 items=["TECH4.00", "TECH7.00", "TECH10.00", "NIST1.68", "NIST4.01", "NIST6.86", "NIST9.18", "NIST12.68"] ("标液2")
                n159 = local write "三点标液3"(w306) -> ()
                n160 = local write "三点标液2"(w307) -> ()
                n161 = local write "三点标液1"(w305) -> ()
              }
              frame 4 {
                w308 = u16 4 items=["TECH4.00", "TECH7.00", "TECH10.00", "NIST1.68", "NIST4.01", "NIST6.86", "NIST9.18", "NIST12.68"] ("标液2")
                w309 = u16 6 items=["TECH4.00", "TECH7.00", "TECH10.00", "NIST1.68", "NIST4.01", "NIST6.86", "NIST9.18", "NIST12.68"] ("标液3")
                w310 = u16 5 items=["TECH4.00", "TECH7.00", "TECH10.00", "NIST1.68", "NIST4.01", "NIST6.86", "NIST9.18", "NIST12.68"] ("标液2")
                n162 = local write "三点标液3"(w309) -> ()
                n163 = local write "三点标液2"(w310) -> ()
                n164 = local write "三点标液1"(w308) -> ()
              }
              frame 5..7 {
                w311 = u16 5 items=["TECH4.00", "TECH7.00", "TECH10.00", "NIST1.68", "NIST4.01", "NIST6.86", "NIST9.18", "NIST12.68"] ("标液2")
                w312 = u16 7 items=["TECH4.00", "TECH7.00", "TECH10.00", "NIST1.68", "NIST4.01", "NIST6.86", "NIST9.18", "NIST12.68"] ("标液3")
                w313 = u16 6 items=["TECH4.00", "TECH7.00", "TECH10.00", "NIST1.68", "NIST4.01", "NIST6.86", "NIST9.18", "NIST12.68"] ("标液2")
                n165 = local write "三点标液3"(w312) -> ()
                n166 = local write "三点标液2"(w313) -> ()
                n167 = local write "三点标液1"(w311) -> ()
              }
            }
            n168 = call "Add State to Queue.vi"("State(s) In (\"\")"=w292) -> ("States Out"=w293:string)  [unwired: 14 in]
          }
          event "三点标液2": Value Change {
            n169 = event-data() -> ("NewVal"=w317:u16)  [unwired: 1 in, 5 out]
            n170 = case shown="6, 7" w317 {
              frame 0..2, Default {
                w318 = u16 0 items=["TECH4.00", "TECH7.00", "TECH10.00", "NIST1.68", "NIST4.01", "NIST6.86", "NIST9.18", "NIST12.68"] ("标液2")
                w319 = u16 2 items=["TECH4.00", "TECH7.00", "TECH10.00", "NIST1.68", "NIST4.01", "NIST6.86", "NIST9.18", "NIST12.68"] ("标液3")
                w320 = u16 1 items=["TECH4.00", "TECH7.00", "TECH10.00", "NIST1.68", "NIST4.01", "NIST6.86", "NIST9.18", "NIST12.68"] ("标液2")
                n171 = local write "三点标液3"(w319) -> ()
                n172 = local write "三点标液2"(w320) -> ()
                n173 = local write "三点标液1"(w318) -> ()
              }
              frame 3, 4 {
                w321 = u16 3 items=["TECH4.00", "TECH7.00", "TECH10.00", "NIST1.68", "NIST4.01", "NIST6.86", "NIST9.18", "NIST12.68"] ("标液2")
                w322 = u16 5 items=["TECH4.00", "TECH7.00", "TECH10.00", "NIST1.68", "NIST4.01", "NIST6.86", "NIST9.18", "NIST12.68"] ("标液3")
                w323 = u16 4 items=["TECH4.00", "TECH7.00", "TECH10.00", "NIST1.68", "NIST4.01", "NIST6.86", "NIST9.18", "NIST12.68"] ("标液2")
                n174 = local write "三点标液3"(w322) -> ()
                n175 = local write "三点标液2"(w323) -> ()
                n176 = local write "三点标液1"(w321) -> ()
              }
              frame 5 {
                w324 = u16 6 items=["TECH4.00", "TECH7.00", "TECH10.00", "NIST1.68", "NIST4.01", "NIST6.86", "NIST9.18", "NIST12.68"] ("标液3")
                w325 = u16 5 items=["TECH4.00", "TECH7.00", "TECH10.00", "NIST1.68", "NIST4.01", "NIST6.86", "NIST9.18", "NIST12.68"] ("标液2")
                n177 = local write "三点标液3"(w324) -> ()
                n178 = local write "三点标液2"(w325) -> ()
              }
              frame 6, 7 {
                w326 = u16 7 items=["TECH4.00", "TECH7.00", "TECH10.00", "NIST1.68", "NIST4.01", "NIST6.86", "NIST9.18", "NIST12.68"] ("标液3")
                w327 = u16 6 items=["TECH4.00", "TECH7.00", "TECH10.00", "NIST1.68", "NIST4.01", "NIST6.86", "NIST9.18", "NIST12.68"] ("标液2")
                n179 = local write "三点标液3"(w326) -> ()
                n180 = local write "三点标液2"(w327) -> ()
              }
            }
            n181 = call "Add State to Queue.vi"("State(s) In (\"\")"=w314) -> ("States Out"=w315:string)  [unwired: 14 in]
          }
          event "三点标液3": Value Change {
            n182 = event-data() -> ("NewVal"=w331:u16)  [unwired: 1 in, 5 out]
            n183 = case shown="3..7" w331 {
              frame 0, 1, Default {
                w332 = u16 2 items=["TECH4.00", "TECH7.00", "TECH10.00", "NIST1.68", "NIST4.01", "NIST6.86", "NIST9.18", "NIST12.68"] ("标液2")
                w333 = u16 0 items=["TECH4.00", "TECH7.00", "TECH10.00", "NIST1.68", "NIST4.01", "NIST6.86", "NIST9.18", "NIST12.68"] ("标液3")
                w334 = u16 1 items=["TECH4.00", "TECH7.00", "TECH10.00", "NIST1.68", "NIST4.01", "NIST6.86", "NIST9.18", "NIST12.68"] ("标液2")
                n184 = local write "三点标液3"(w333) -> ()
                n185 = local write "三点标液2"(w334) -> ()
                n186 = local write "三点标液1"(w332) -> ()
              }
              frame 2 {
                w335 = u16 0 items=["TECH4.00", "TECH7.00", "TECH10.00", "NIST1.68", "NIST4.01", "NIST6.86", "NIST9.18", "NIST12.68"] ("标液2")
                w336 = u16 2 items=["TECH4.00", "TECH7.00", "TECH10.00", "NIST1.68", "NIST4.01", "NIST6.86", "NIST9.18", "NIST12.68"] ("标液3")
                w337 = u16 1 items=["TECH4.00", "TECH7.00", "TECH10.00", "NIST1.68", "NIST4.01", "NIST6.86", "NIST9.18", "NIST12.68"] ("标液2")
                n187 = local write "三点标液3"(w336) -> ()
                n188 = local write "三点标液2"(w337) -> ()
                n189 = local write "三点标液1"(w335) -> ()
              }
              frame 3..7 {
                n190 = local read "三点标液1"() -> (w340:u16)
                n191 = local read "三点标液2"() -> (w339:u16)
                n192 = Less?(x=w340, y=w339) -> (x < y?=w338:bool)
                n193 = case shown="假" w338 {
                  frame False {
                  }
                  frame True {
                    n194 = local read "三点标液3"() -> (w343:u16)
                    n195 = local read "三点标液2"() -> (w341:u16)
                    n196 = Less Or Equal?(x=w343, y=w341) -> (x <= y?=w342:bool)
                    n197 = case shown="真" w342 {
                      tunnel: w341 -> [_ w345]
                      frame False {
                      }
                      frame True {
                        n198 = Increment(x=w345) -> (x+1=w344:u16)
                        n199 = local write "三点标液3"(w344) -> ()
                      }
                    }
                  }
                }
              }
            }
            n200 = call "Add State to Queue.vi"("State(s) In (\"\")"=w328) -> ("States Out"=w329:string)  [unwired: 14 in]
          }
          event "标液1", "标液2", "偏移值补偿": Mouse Down {
            n201 = event-data() -> ("CtlRef"=w350:refnum<vi>)  [unwired: 1 in, 7 out]
            n202 = property on="校准模式" class="Ring (严格)"() -> ("DisabledEnum"=w348:T3)  [unwired: 2 in, 2 out]
            n203 = case shown="\"Enabled\"" w348 {
              tunnel: w350 -> [w354 _]
              frame "Enabled" {
                n204 = property class="DigNum (严格)"(reference=w354) -> (reference out=w351:refnum<vi>, "Value"=w352:dbl)  [unwired: 1 in, 1 out]
                n205 = call "数字键盘.vi"("OldNumber"=w352) -> ("NewNumber"=w353:dbl)  [unwired: 1 in]
                n206 = property class="DigNum (严格)"(reference=w351, "Val(Sgnl)"=w353) -> ()  [unwired: 1 in, 2 out]
              }
              frame "Disabled", Default {
              }
            }
            n207 = call "Add State to Queue.vi"("State(s) In (\"\")"=w346) -> ("States Out"=w347:string)  [unwired: 14 in]
          }
          event "偏移值补偿": Value Change {
            n208 = event-data() -> ("NewVal"=w356:dbl)  [unwired: 1 in, 5 out]
            n209 = global read "多参数全局变量.vi" "MB session in"() -> (w357:refnum<class "MB_Master.lvclass">)
            n210 = call "000CH_pH_pH偏移修正值写入.vi"("数值"=w356, "MB session in"=w357) -> ("error out"=w355:errorcluster)  [unwired: 8 in, 1 out]
            n211 = call "Add State to Queue.vi"("State(s) In (\"\")"=w360) -> ("States Out"=w359:string)  [unwired: 14 in]
          }
          event "标液1": Value Change {
            n212 = event-data() -> ("NewVal"=w366:dbl)  [unwired: 1 in, 5 out]
            n213 = global read "多参数全局变量.vi" "MB session in"() -> (w364:refnum<class "MB_Master.lvclass">)
            n214 = call "0030H_pH_第一点标准值写入.vi"("数值"=w366, "MB session in"=w364) -> ("error out"=w365:errorcluster)  [unwired: 8 in, 1 out]
            n215 = call "Add State to Queue.vi"("State(s) In (\"\")"=w361) -> ("States Out"=w362:string)  [unwired: 14 in]
          }
          event "标液2": Value Change {
            n216 = event-data() -> ("NewVal"=w372:dbl)  [unwired: 1 in, 5 out]
            n217 = global read "多参数全局变量.vi" "MB session in"() -> (w370:refnum<class "MB_Master.lvclass">)
            n218 = call "Add State to Queue.vi"("State(s) In (\"\")"=w367) -> ("States Out"=w368:string)  [unwired: 14 in]
            n219 = call "0033H_pH_第二点标准值写入.vi"("数值"=w372, "MB session in"=w370) -> ("error out"=w371:errorcluster)  [unwired: 8 in, 1 out]
          }
          event "刷新按钮": Value Change {
            n220 = event-data() -> ()  [unwired: 1 in, 6 out]
            n221 = call "Add State to Queue.vi"("State(s) In (\"\")"=w375) -> ("States Out"=w374:string)  [unwired: 14 in]
            n222 = Two Button Dialog(message="请再次确实是否恢复出厂设置！" ("消息")) -> (T button?=w377:bool)  [unwired: 2 in]
            n223 = case shown="真" w377 {
              frame False {
              }
              frame True {
                w378 = u16 33 items=["Factory Reset"=33] ("数值")
                n224 = global read "多参数全局变量.vi" "MB session in"() -> (w379:refnum<class "MB_Master.lvclass">)
                n225 = call "0026H_pH_命令寄存器写入.vi"("数值"=w378, "MB session in"=w379) -> ()  [unwired: 8 in, 2 out]
              }
            }
          }
          event "校准启动": Value Change {
            n226 = event-data() -> ()  [unwired: 1 in, 6 out]
            n227 = global read "多参数全局变量.vi" "校准运行状态"() -> (w381:T4)
            n228 = Bundle By Name(cluster=w381, "ph"=TRUE) -> (w382:T4)
            n229 = call "Add State to Queue.vi"("State(s) In (\"\")"=w386, "State(s) At Back (\"\")"="init: all\nCal: Place standard solution\n Cal: Calibration process\nidle" ("State(s) In (\"\")")) -> ("States Out"=w385:string)  [unwired: 13 in]
            n230 = global write "多参数全局变量.vi" "校准运行状态"(w382) -> ()
          }
          event "校准停止": Value Change {
            n231 = event-data() -> ()  [unwired: 1 in, 6 out]
            n232 = call "Add State to Queue.vi"("State(s) In (\"\")"="init: all\nCal: Over\nidle" ("State(s) In (\"\")")) -> ("States Out"=w388:string)  [unwired: 14 in]
          }
        }
      }
    }
  }
  n233 = while {
    stop <- FALSE stop-if-true
    n234 = global read "多参数全局变量.vi" "权限"() -> (w393:enum16{"一级权限", "二级权限", "三级权限"})
    n235 = Wait (ms)(milliseconds to wait=u32 1000 ("等待时间（毫秒）")) -> ()  [unwired: 1 out]
    n236 = Not Equal?(x=w393, y=enum16{"一级权限", "二级权限", "三级权限"}."一级权限") -> (x != y?=w391:bool)
    n237 = property on="偏移值补偿" class="DigNum (严格)"("Visible"=w391) -> ()  [unwired: 2 in, 2 out]
  }
